vi "Test50_micro.vi"(9 "SN":string, 10 "Out":T1) -> (3 "String":string)   [LabVIEW 2020]
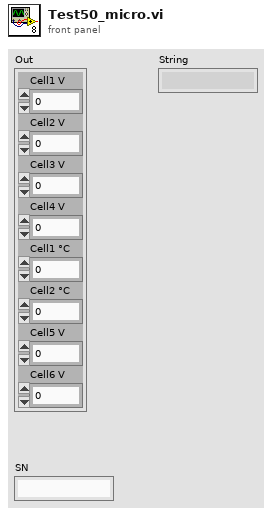
[diagram p1: front panel]
types:
  T1 = cluster{"Cell1 V":sgl, "Cell2 V":sgl, "Cell3 V":sgl, "Cell4 V":sgl, "Cell1 °C":sgl, "Cell2 °C":sgl, "Cell5 V":sgl, "Cell6 V":sgl}
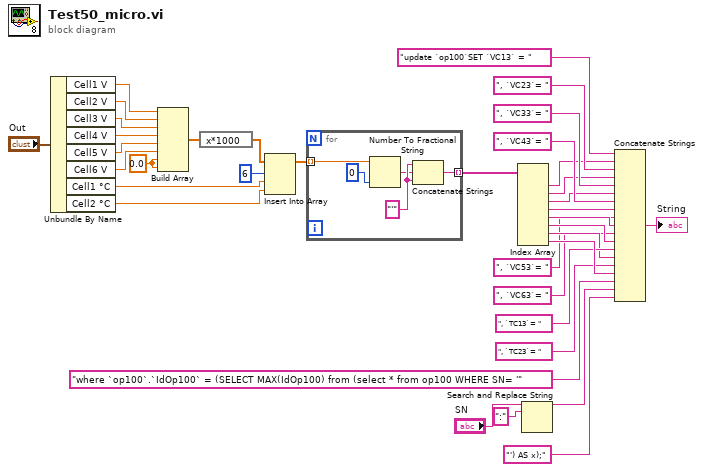
[diagram p0: block diagram]
diagram:
  w14 = sgl 0.0 ("élément")
  n1 = Unbundle By Name("Out") -> ("Cell1 V"=w12:sgl, "Cell2 V"=w11:sgl, "Cell3 V"=w10:sgl, "Cell4 V"=w9:sgl, "Cell5 V"=w8:sgl, "Cell6 V"=w7:sgl, "Cell1 °C"=w3:sgl, "Cell2 °C"=w2:sgl)
  n2 = Build Array(w12, w11, w10, w9, w8, w7, w14, w14) -> (w6:sgl[])
  n3 = expression code="x*1000"(w6) -> (w5:sgl[])
  n4 = Insert Into Array(array=w5, index=6 ("indice"), new element #1=w3, new element #2=w2) -> (w1:sgl[])
  n5 = for {
    tunnel: w1 -> [w42] mode=indexing
    tunnel: [w39] -> w20 mode=indexing
    w40 = "'" ("chaîne")
    n6 = Number To Fractional String ("Nombre en chaîne fractionnaire")(number=w42, precision (6)=i16 0 ("précision (6)")) -> (F-format string=w38:string)  [unwired: 2 in]
    n7 = Concatenate Strings(w40, w38, w40) -> (w39:string)
  }
  n8 = Index Array(array=w20) -> (element #1=w21:string, element #2=w23:string, element #3=w25:string, element #4=w27:string, element #5=w29:string, element #6=w31:string, element #7=w32:string, element #8=w35:string)  [unwired: 8 in]
  n9 = Search and Replace String ("Rechercher et remplacer une chaîne")(input string="SN", search string=":" ("chaîne recherchée")) -> (result string=w18:string)  [unwired: 6 in, 3 out]
  n10 = Concatenate Strings("update `op100`SET `VC13` = " ("chaîne"), w21, ", `VC23`= " ("chaîne"), w23, ", `VC33`= " ("chaîne"), w25, ", `VC43`= " ("chaîne"), w27, ", `VC53`= " ("chaîne"), w29, ", `VC63`= " ("chaîne"), w31, ", `TC13`= " ("chaîne"), w32, ", `TC23`= " ("chaîne"), w35, "where `op100`.`IdOp100` = (SELECT MAX(IdOp100) from (select * from op100 WHERE SN= '" ("chaîne"), w18, "') AS x);" ("chaîne")) -> (→"String":string)
